vi "Measure Y verses voltage.vi"() -> ()   [LabVIEW 2020]
uses:
  <vilib>/DAQmx/write.llb/DAQmx Write (Analog 2D DBL NChan NSamp).vi
  <vilib>/DAQmx/create/channels.llb/DAQmx Create Channel (AO-Voltage-Basic).vi
  <vilib>/DAQmx/configure/timing.llb/DAQmx Timing (Use Waveform).vi
  <vilib>/Utility/file.llb/Write Delimited Spreadsheet (DBL).vi
  <vilib>/DAQmx/miscellaneous.llb/DAQmx Fill In Error Info.vi
  <vilib>/measure/NI_MABase.lvlib
panel:
  out "x+y":dbl=491.0
  in  "Voltage value at top of FOV":dbl=0.207
  out "dt":dbl=10.0
  out "Voice coil response (blue) 2":dbl[][](graph)=[[-0.284, -0.27908999999999995, -0.27418, -0.26927, -0.26436000000000004, -0.25945, -0.25454, -0.24963, -0.24472, -0.23981, -0.2349, -0.22999, -0.22507999999999997, -0.22017, -0.21525999999999998, -0.21034999999999998, -0.20544, -0.20053, -0.19562000000000002, -0.19071, -0.18580000000000002, -0.18089, -0.17598, -0.17107, -0.16616, -0.16125, -0.15634, -0.15143, -0.14651999999999998, -0.14160999999999999, -0.1367, -0.13179, -0.12688, -0.12197, -0.11706, -0.11215, -0.10724000000000002, -0.10232999999999999, -0.09741999999999999, -0.09251, -0.0876, -0.08269, -0.07778, -0.07287, -0.06795999999999998, -0.06304999999999998, -0.05813999999999998, -0.05322999999999999, -0.048319999999999995, -0.04341, -0.0385, -0.03359, -0.028680000000000008, -0.023769999999999982, -0.018860000000000012, -0.013949999999999988, -0.009039999999999963, -0.004129999999999996, 0.0007800000000000296, 0.005689999999999998, 0.010600000000000023, 0.01550999999999999, 0.020420000000000015, 0.025329999999999984, 0.03024000000000001, 0.035150000000000035, 0.040060000000000005, 0.044970000000000024, 0.049879999999999994, 0.05479000000000002, 0.05969999999999999, 0.06461000000000001, 0.06951999999999998, 0.07443000000000001, 0.07934000000000004, 0.08425, 0.08916000000000003, 0.09406999999999999, 0.09898000000000001, 0.10388999999999998, 0.10880000000000001, 0.11371000000000003, 0.11862, 0.12353000000000003, 0.12844, 0.13335000000000002, 0.13826, 0.14317000000000002, 0.14808000000000004, 0.15299000000000001, 0.15790000000000004, 0.16281, 0.16772000000000004, 0.17263, 0.17754000000000003, 0.18245, 0.18736000000000003, 0.19227000000000005, 0.19718, 0.20209000000000002, 0.207, 0.0, 0.0, 0.0, 0.0, 0.0, 0.0, 0.0, 0.0, 0.0, 0.0, 0.0, 0.0, 0.0, 0.0, 0.0, 0.0, 0.0, 0.0, 0.0, 0.0, 0.0, 0.0, 0.0, 0.0, 0.0, 0.0, 0.0, 0.0, 0.0, 0.0, 0.0, 0.0, 0.0, 0.0, 0.0, 0.0, 0.0, 0.0, 0.0, 0.0, 0.0, 0.0, 0.0, 0.0, 0.0, 0.0, 0.0, 0.0, 0.0, 0.0, 0.0, 0.0, 0.0, 0.0, 0.0, 0.0, 0.0, 0.0, 0.0, 0.0, 0.0, 0.0, 0.0, 0.0, 0.0, 0.0, 0.0, 0.0, 0.0, 0.0, 0.0, 0.0, 0.0, 0.0, 0.0, 0.0, 0.0, 0.0, 0.0, 0.0, 0.0, 0.0, 0.0, 0.0, 0.0, 0.0, 0.0, 0.0, 0.0, 0.0, 0.0, 0.0, 0.0, 0.0, 0.0, 0.0, 0.0, 0.0, 0.0, 0.0, 0.0, 0.0, 0.0, 0.0, 0.0, 0.0, 0.0, 0.0, 0.0, 0.0, 0.0, 0.0, 0.0, 0.0, 0.0, 0.0, 0.0, 0.0, 0.0, 0.0, 0.0, 0.0, 0.0, 0.0, 0.0, 0.0, 0.0, 0.0, 0.0, 0.0, 0.0, 0.0, 0.0, 0.0, 0.0, 0.0, 0.0, 0.0, 0.0, 0.0, 0.0, 0.0, 0.0, 0.0, 0.0, 0.0, 0.0, 0.0, 0.0, 0.0, 0.0, 0.0, 0.0, 0.0, 0.0, 0.0, 0.0, 0.0, 0.0, 0.0, 0.0, 0.0, 0.0, 0.0, 0.0, 0.0, 0.0, 0.0, 0.0, 0.0, 0.0, 0.0, 0.0, 0.0, 0.0, 0.0, 0.0, 0.0, 0.0, 0.0, 0.0, 0.0, 0.0, 0.0, 0.0, 0.0, 0.0, 0.0, 0.0, 0.0, 0.0, 0.0, 0.0, 0.0, 0.0, 0.0, 0.0, 0.0, 0.0, 0.0, 0.0, 0.0, 0.0, 0.0, 0.0, 0.0, 0.0, 0.0, 0.0, 0.0, 0.0, 0.0, 0.0, 0.0, 0.0, 0.0, 0.0, 0.0, 0.0, 0.0, 0.0, 0.0, 0.0, 0.0, 0.0, 0.0, 0.0, 0.0, 0.0, 0.0, 0.0, 0.0, 0.0, 0.0, 0.0, 0.0, 0.0, 0.0, 0.0, 0.0, 0.0, 0.0, 0.0, 0.0, 0.0, 0.0, 0.0, 0.0, 0.0, 0.0, 0.0, 0.0, 0.0, 0.0, 0.0, 0.0, 0.0, 0.0, 0.0, 0.0, 0.0, 0.0, 0.0, 0.0, 0.0, 0.0, 0.0, 0.0, 0.0, 0.0, 0.0, 0.0, 0.0, 0.0, 0.0, 0.0, 0.0, 0.0, 0.0, 0.0, 0.0, 0.0, 0.0, 0.0, 0.0, 0.0, 0.0, 0.0, 0.0, 0.0, 0.0, 0.0, 0.0, 0.0, 0.0, 0.0, 0.0, 0.0, 0.0, 0.0, 0.0, 0.0, 0.0, 0.0, 0.0, 0.0, 0.0, 0.0, 0.0, 0.0, 0.0, 0.0, 0.0, 0.0, 0.0, 0.0, 0.0, 0.0, 0.0, 0.0, 0.0, 0.0, 0.0, 0.0, 0.0, 0.0, 0.0, 0.0, 0.0, 0.0, 0.0, 0.0, 0.0, 0.0, 0.0, 0.0, 0.0, 0.0, 0.0, 0.0, 0.0, 0.0, 0.0, 0.0, 0.0, 0.0, 0.0, 0.0, 0.0, 0.0, 0.0, 0.0, 0.0, 0.0, 0.0, 0.0, 0.0, 0.0, 0.0, 0.0, 0.0, 0.0, 0.0, 0.0, 0.0, 0.0, 0.0, 0.0, 0.0, 0.0, 0.0, 0.0, 0.0, 0.0, 0.0, 0.0, 0.0, 0.0, 0.0, 0.0, 0.0, 0.0, 0.0, 0.0, 0.0, 0.0, 0.0, 0.0, 0.0, 0.0, 0.0, 0.0, 0.0, 0.0, 0.0, 0.0, 0.0, 0.0, 0.0, 0.0, 0.0, 0.0, 0.0, 0.0, 0.0, 0.0, 0.0, 0.0, 0.0, 0.0, 0.0, 0.0, 0.0, 0.0, 0.0, 0.0, 0.0, 0.0, 0.0, 0.0, 0.0, 0.0, 0.0, 0.0, 0.0, 0.0, 0.0, 0.0, 0.0, 0.0, 0.0, 0.0, 0.0, 0.0, 0.0, 0.0, 0.0, 0.0, 0.0, 0.0, 0.0, 0.0, 0.0, 0.0, 0.0, 0.0, 0.0, 0.0, 0.0, 0.0, 0.0, 0.0, 0.0, 0.0, 0.0, 0.0, 0.0, 0.0, 0.0, 0.0, 0.0, 0.0, 0.0, 0.0, 0.0, 0.0, 0.0, 0.0, 0.0, 0.0, 0.0, 0.0, 0.0, 0.0, 0.0, 0.0, 0.0, 0.0, 0.0, 0.0, 0.0, 0.0, 0.0, 0.0, 0.0, 0.0, 0.0, 0.0, 0.0, 0.0, 0.0, 0.0, 0.0, 0.0, 0.0, 0.0, 0.0, 0.0, 0.0, 0.0, 0.0, 0.0, 0.0, 0.0, 0.0, 0.0, 0.0, 0.0, 0.0, 0.0, 0.0, 0.0, 0.0, 0.0, 0.0, 0.0, 0.0, 0.0, 0.0, 0.0, 0.0, 0.0, 0.0, 0.0, 0.0, 0.0, 0.0, 0.0, 0.0, 0.0, 0.0, 0.0, 0.0, 0.0, 0.0, 0.0, 0.0, 0.0, 0.0, 0.0, 0.0, 0.0, 0.0, 0.0, 0.0, 0.0, 0.0, 0.0, 0.0, 0.0, 0.0, 0.0, 0.0, 0.0, 0.0, 0.0, 0.0, 0.0, 0.0, 0.0, 0.0, 0.0, 0.0, 0.0, 0.0, 0.0, 0.0, 0.0, 0.0, 0.0, 0.0, 0.0, 0.0, 0.0, 0.0, 0.0, 0.0, 0.0, 0.0, 0.0, 0.0, 0.0, 0.0, 0.0, 0.0, 0.0, 0.0, 0.0, 0.0, 0.0, 0.0, 0.0, 0.0, 0.0, 0.0, 0.0, 0.0, 0.0, 0.0, 0.0, 0.0, 0.0, 0.0, 0.0, 0.0, 0.0, 0.0, 0.0, 0.0, 0.0, 0.0, 0.0, 0.0, 0.0, 0.0, 0.0, 0.0, 0.0, 0.0, 0.0, 0.0, 0.0, 0.0, 0.0, 0.0, 0.0, 0.0, 0.0, 0.0, 0.0, 0.0, 0.0, 0.0, 0.0, 0.0, 0.0, 0.0, 0.0, 0.0, 0.0, 0.0, 0.0, 0.0, 0.0, 0.0, 0.0, 0.0, 0.0, 0.0, 0.0, 0.0, 0.0, 0.0, 0.0, 0.0, 0.0, 0.0, 0.0, 0.0, 0.0, 0.0, 0.0, 0.0, 0.0, 0.0, 0.0, 0.0, 0.0, 0.0, 0.0, 0.0, 0.0, 0.0, 0.0, 0.0, 0.0, 0.0, 0.0, 0.0, 0.0, 0.0, 0.0, 0.0, 0.0, 0.0, 0.0, 0.0, 0.0, 0.0, 0.0, 0.0, 0.0, 0.0, 0.0, 0.0, 0.0, 0.0, 0.0, 0.0, 0.0, 0.0, 0.0, 0.0, 0.0, 0.0, 0.0, 0.0, 0.0, 0.0, 0.0, 0.0, 0.0, 0.0, 0.0, 0.0, 0.0, 0.0, 0.0, 0.0, 0.0, 0.0, 0.0, 0.0, 0.0, 0.0, 0.0, 0.0, 0.0, 0.0, 0.0, 0.0, 0.0, 0.0, 0.0, 0.0, 0.0, 0.0, 0.0, 0.0, 0.0, 0.0, 0.0, 0.0, 0.0, 0.0, 0.0, 0.0, 0.0, 0.0, 0.0, 0.0, 0.0, 0.0, 0.0, 0.0, 0.0, 0.0, 0.0, 0.0, 0.0, 0.0, 0.0, 0.0, 0.0, 0.0, 0.0, 0.0, 0.0, 0.0, 0.0, 0.0, 0.0, 0.0, 0.0, 0.0, 0.0, 0.0, 0.0, 0.0, 0.0, 0.0, 0.0, 0.0, 0.0, 0.0, 0.0, 0.0, 0.0, 0.0, 0.0, 0.0, 0.0, 0.0, 0.0, 0.0, 0.0, 0.0, 0.0, 0.0, 0.0, 0.0, 0.0, 0.0, 0.0, 0.0, 0.0, 0.0, 0.0, 0.0, 0.0, 0.0, 0.0, 0.0, 0.0, 0.0, 0.0, 0.0, 0.0, 0.0, 0.0, 0.0, 0.0, 0.0, 0.0, 0.0, 0.0, 0.0, 0.0, 0.0, 0.0, 0.0, 0.0, 0.0, 0.0, 0.0, 0.0, 0.0, 0.0, 0.0, 0.0, 0.0, 0.0, 0.0, 0.0, 0.0, 0.0, 0.0, 0.0, 0.0, 0.0, 0.0, 0.0, 0.0, 0.0, 0.0, 0.0, 0.0, 0.0, 0.0, 0.0, 0.0, 0.0, 0.0, 0.0, 0.0, 0.0, 0.0, 0.0, 0.0, 0.0, 0.0, 0.0, 0.0, 0.0, 0.0, 0.0, 0.0, 0.0, 0.0, 0.0, 0.0, 0.0, 0.0, 0.0, 0.0, 0.0, 0.0, 0.0, 0.0, 0.0, 0.0, 0.0, 0.0, 0.0, 0.0, 0.0, 0.0, 0.0, 0.0], [0.0, 5.0, 0.0, 5.0, 0.0, 5.0, 0.0, 5.0, 0.0, 5.0, 0.0, 5.0, 0.0, 5.0, 0.0, 5.0, 0.0, 5.0, 0.0, 5.0, 0.0, 5.0, 0.0, 5.0, 0.0, 5.0, 0.0, 5.0, 0.0, 5.0, 0.0, 5.0, 0.0, 5.0, 0.0, 5.0, 0.0, 5.0, 0.0, 5.0, 0.0, 5.0, 0.0, 5.0, 0.0, 5.0, 0.0, 5.0, 0.0, 5.0, 0.0, 5.0, 0.0, 5.0, 0.0, 5.0, 0.0, 5.0, 0.0, 5.0, 0.0, 5.0, 0.0, 5.0, 0.0, 5.0, 0.0, 5.0, 0.0, 5.0, 0.0, 5.0, 0.0, 5.0, 0.0, 5.0, 0.0, 5.0, 0.0, 5.0, 0.0, 5.0, 0.0, 5.0, 0.0, 5.0, 0.0, 5.0, 0.0, 5.0, 0.0, 5.0, 0.0, 5.0, 0.0, 5.0, 0.0, 5.0, 0.0, 5.0, 0.0, 5.0, 0.0, 5.0, 0.0, 5.0, 0.0, 5.0, 0.0, 5.0, 0.0, 5.0, 0.0, 5.0, 0.0, 5.0, 0.0, 5.0, 0.0, 5.0, 0.0, 5.0, 0.0, 5.0, 0.0, 5.0, 0.0, 5.0, 0.0, 5.0, 0.0, 5.0, 0.0, 5.0, 0.0, 5.0, 0.0, 5.0, 0.0, 5.0, 0.0, 5.0, 0.0, 5.0, 0.0, 5.0, 0.0, 5.0, 0.0, 5.0, 0.0, 5.0, 0.0, 5.0, 0.0, 5.0, 0.0, 5.0, 0.0, 5.0, 0.0, 5.0, 0.0, 5.0, 0.0, 5.0, 0.0, 5.0, 0.0, 5.0, 0.0, 5.0, 0.0, 5.0, 0.0, 5.0, 0.0, 5.0, 0.0, 5.0, 0.0, 5.0, 0.0, 5.0, 0.0, 5.0, 0.0, 5.0, 0.0, 5.0, 0.0, 5.0, 0.0, 5.0, 0.0, 5.0, 0.0, 5.0, 0.0, 5.0, 0.0, 5.0, 0.0, 5.0, 0.0, 5.0, 0.0, 5.0, 0.0, 5.0, 0.0, 5.0, 0.0, 5.0, 0.0, 5.0, 0.0, 5.0, 0.0, 5.0, 0.0, 5.0, 0.0, 5.0, 0.0, 5.0, 0.0, 5.0, 0.0, 5.0, 0.0, 5.0, 0.0, 5.0, 0.0, 5.0, 0.0, 5.0, 0.0, 5.0, 0.0, 5.0, 0.0, 5.0, 0.0, 5.0, 0.0, 5.0, 0.0, 5.0, 0.0, 5.0, 0.0, 5.0, 0.0, 5.0, 0.0, 5.0, 0.0, 5.0, 0.0, 5.0, 0.0, 5.0, 0.0, 5.0, 0.0, 5.0, 0.0, 5.0, 0.0, 5.0, 0.0, 5.0, 0.0, 5.0, 0.0, 5.0, 0.0, 5.0, 0.0, 5.0, 0.0, 5.0, 0.0, 5.0, 0.0, 5.0, 0.0, 5.0, 0.0, 5.0, 0.0, 5.0, 0.0, 5.0, 0.0, 5.0, 0.0, 5.0, 0.0, 5.0, 0.0, 5.0, 0.0, 5.0, 0.0, 5.0, 0.0, 5.0, 0.0, 5.0, 0.0, 5.0, 0.0, 5.0, 0.0, 5.0, 0.0, 5.0, 0.0, 5.0, 0.0, 5.0, 0.0, 5.0, 0.0, 5.0, 0.0, 5.0, 0.0, 5.0, 0.0, 5.0, 0.0, 5.0, 0.0, 5.0, 0.0, 5.0, 0.0, 5.0, 0.0, 5.0, 0.0, 5.0, 0.0, 5.0, 0.0, 5.0, 0.0, 5.0, 0.0, 5.0, 0.0, 5.0, 0.0, 5.0, 0.0, 5.0, 0.0, 5.0, 0.0, 5.0, 0.0, 5.0, 0.0, 5.0, 0.0, 5.0, 0.0, 5.0, 0.0, 5.0, 0.0, 5.0, 0.0, 5.0, 0.0, 5.0, 0.0, 5.0, 0.0, 5.0, 0.0, 5.0, 0.0, 5.0, 0.0, 5.0, 0.0, 5.0, 0.0, 5.0, 0.0, 5.0, 0.0, 5.0, 0.0, 5.0, 0.0, 5.0, 0.0, 5.0, 0.0, 5.0, 0.0, 5.0, 0.0, 5.0, 0.0, 5.0, 0.0, 5.0, 0.0, 5.0, 0.0, 5.0, 0.0, 5.0, 0.0, 5.0, 0.0, 5.0, 0.0, 5.0, 0.0, 5.0, 0.0, 5.0, 0.0, 5.0, 0.0, 5.0, 0.0, 5.0, 0.0, 5.0, 0.0, 5.0, 0.0, 5.0, 0.0, 5.0, 0.0, 5.0, 0.0, 5.0, 0.0, 5.0, 0.0, 5.0, 0.0, 5.0, 0.0, 5.0, 0.0, 5.0, 0.0, 5.0, 0.0, 5.0, 0.0, 5.0, 0.0, 5.0, 0.0, 5.0, 0.0, 5.0, 0.0, 5.0, 0.0, 5.0, 0.0, 5.0, 0.0, 5.0, 0.0, 5.0, 0.0, 5.0, 0.0, 5.0, 0.0, 5.0, 0.0, 5.0, 0.0, 5.0, 0.0, 5.0, 0.0, 5.0, 0.0, 5.0, 0.0, 5.0, 0.0, 5.0, 0.0, 5.0, 0.0, 5.0, 0.0, 5.0, 0.0, 5.0, 0.0, 5.0, 0.0, 5.0, 0.0, 5.0, 0.0, 5.0, 0.0, 5.0, 0.0, 5.0, 0.0, 5.0, 0.0, 5.0, 0.0, 5.0, 0.0, 5.0, 0.0, 5.0, 0.0, 5.0, 0.0, 5.0, 0.0, 5.0, 0.0, 5.0, 0.0, 5.0, 0.0, 5.0, 0.0, 5.0, 0.0, 5.0, 0.0, 5.0, 0.0, 5.0, 0.0, 5.0, 0.0, 5.0, 0.0, 5.0, 0.0, 5.0, 0.0, 5.0, 0.0, 5.0, 0.0, 5.0, 0.0, 5.0, 0.0, 5.0, 0.0, 5.0, 0.0, 5.0, 0.0, 5.0, 0.0, 5.0, 0.0, 5.0, 0.0, 5.0, 0.0, 5.0, 0.0, 5.0, 0.0, 5.0, 0.0, 5.0, 0.0, 5.0, 0.0, 5.0, 0.0, 5.0, 0.0, 5.0, 0.0, 5.0, 0.0, 5.0, 0.0, 5.0, 0.0, 5.0, 0.0, 5.0, 0.0, 5.0, 0.0, 5.0, 0.0, 5.0, 0.0, 5.0, 0.0, 5.0, 0.0, 5.0, 0.0, 5.0, 0.0, 5.0, 0.0, 5.0, 0.0, 5.0, 0.0, 5.0, 0.0, 5.0, 0.0, 5.0, 0.0, 5.0, 0.0, 5.0, 0.0, 5.0, 0.0, 5.0, 0.0, 5.0, 0.0, 5.0, 0.0, 5.0, 0.0, 5.0, 0.0, 5.0, 0.0, 5.0, 0.0, 5.0, 0.0, 5.0, 0.0, 5.0, 0.0, 5.0, 0.0, 5.0, 0.0, 5.0, 0.0, 5.0, 0.0, 5.0, 0.0, 5.0, 0.0, 5.0, 0.0, 5.0, 0.0, 5.0, 0.0, 5.0, 0.0, 5.0, 0.0, 5.0, 0.0, 5.0, 0.0, 5.0, 0.0, 5.0, 0.0, 5.0, 0.0, 5.0, 0.0, 5.0, 0.0, 5.0, 0.0, 5.0, 0.0, 5.0, 0.0, 5.0, 0.0, 5.0, 0.0, 5.0, 0.0, 5.0, 0.0, 5.0, 0.0, 5.0, 0.0, 5.0, 0.0, 5.0, 0.0, 5.0, 0.0, 5.0, 0.0, 5.0, 0.0, 5.0, 0.0, 5.0, 0.0, 5.0, 0.0, 5.0, 0.0, 5.0, 0.0, 5.0, 0.0, 5.0, 0.0, 5.0, 0.0, 5.0, 0.0, 5.0, 0.0, 5.0, 0.0, 5.0, 0.0, 5.0, 0.0, 5.0, 0.0, 5.0, 0.0, 5.0, 0.0, 5.0, 0.0, 5.0, 0.0, 5.0, 0.0, 5.0, 0.0, 5.0, 0.0, 5.0, 0.0, 5.0, 0.0, 5.0, 0.0, 5.0, 0.0, 5.0, 0.0, 5.0, 0.0, 5.0, 0.0, 5.0, 0.0, 5.0, 0.0, 5.0, 0.0, 5.0, 0.0, 5.0, 0.0, 5.0, 0.0, 5.0, 0.0, 5.0, 0.0, 5.0, 0.0, 5.0, 0.0, 5.0, 0.0, 5.0, 0.0, 5.0, 0.0, 5.0, 0.0, 5.0, 0.0, 5.0, 0.0, 5.0, 0.0, 5.0, 0.0, 5.0, 0.0, 5.0, 0.0, 5.0, 0.0, 5.0, 0.0, 5.0, 0.0, 5.0, 0.0, 5.0, 0.0, 5.0, 0.0, 5.0, 0.0, 5.0, 0.0, 5.0, 0.0, 5.0, 0.0, 5.0, 0.0, 5.0, 0.0, 5.0, 0.0, 5.0, 0.0, 5.0, 0.0, 5.0, 0.0, 5.0, 0.0, 5.0, 0.0, 5.0, 0.0, 5.0, 0.0, 5.0, 0.0, 5.0, 0.0, 5.0, 0.0, 5.0, 0.0, 5.0, 0.0, 5.0, 0.0, 5.0, 0.0, 5.0, 0.0, 5.0, 0.0, 5.0, 0.0, 5.0, 0.0, 5.0, 0.0, 5.0, 0.0, 5.0, 0.0, 5.0, 0.0, 5.0, 0.0, 5.0, 0.0, 5.0, 0.0, 5.0, 0.0, 5.0, 0.0, 5.0, 0.0, 5.0, 0.0, 5.0, 0.0, 5.0, 0.0, 5.0, 0.0, 5.0, 0.0, 5.0, 0.0, 5.0, 0.0, 5.0, 0.0, 5.0, 0.0, 5.0, 0.0, 5.0, 0.0, 5.0, 0.0, 5.0, 0.0, 5.0, 0.0, 5.0, 0.0, 5.0, 0.0, 5.0, 0.0, 5.0, 0.0, 5.0, 0.0, 5.0, 0.0, 5.0, 0.0, 5.0, 0.0, 5.0, 0.0, 5.0, 0.0, 5.0, 0.0, 5.0, 0.0, 5.0, 0.0, 5.0, 0.0, 5.0, 0.0, 5.0, 0.0, 5.0, 0.0, 5.0, 0.0, 5.0, 0.0, 5.0, 0.0, 5.0, 0.0, 5.0, 0.0, 5.0, 0.0, 5.0, 0.0, 5.0, 0.0, 5.0, 0.0, 5.0, 0.0, 5.0, 0.0, 5.0, 0.0, 5.0, 0.0, 5.0, 0.0, 5.0, 0.0, 5.0, 0.0, 5.0, 0.0, 5.0, 0.0, 5.0]]
  out "x/y 2":dbl=0.01
  out "x/y":dbl=4.91
  out "x*y":dbl=491.0
  in  "Number of frames":dbl=100.0
  in  "file path (dialog if empty)":path=path "C:/Users/htm22/Downloads/Voltage positions.txt"
  in  "Voltage value at bottom of FOV":dbl=-0.284
  out "# Samples written per channel":u32=1000
  in  "Stop 2":bool
  out "Maximum Voltage value at top of FOV":dbl=0.207
  out "Voice coil response (blue)":waveform(dbl)[](graph)=[{"t0"=timestamp(0 s since 1904-01-01), "dt"=10.0, "Y"=[-0.284, -0.27908999999999995, -0.27418, -0.26927, -0.26436000000000004, -0.25945, -0.25454, -0.24963, -0.24472, -0.23981, -0.2349, -0.22999, -0.22507999999999997, -0.22017, -0.21525999999999998, -0.21034999999999998, -0.20544, -0.20053, -0.19562000000000002, -0.19071, -0.18580000000000002, -0.18089, -0.17598, -0.17107, -0.16616, -0.16125, -0.15634, -0.15143, -0.14651999999999998, -0.14160999999999999, -0.1367, -0.13179, -0.12688, -0.12197, -0.11706, -0.11215, -0.10724000000000002, -0.10232999999999999, -0.09741999999999999, -0.09251, -0.0876, -0.08269, -0.07778, -0.07287, -0.06795999999999998, -0.06304999999999998, -0.05813999999999998, -0.05322999999999999, -0.048319999999999995, -0.04341, -0.0385, -0.03359, -0.028680000000000008, -0.023769999999999982, -0.018860000000000012, -0.013949999999999988, -0.009039999999999963, -0.004129999999999996, 0.0007800000000000296, 0.005689999999999998, 0.010600000000000023, 0.01550999999999999, 0.020420000000000015, 0.025329999999999984, 0.03024000000000001, 0.035150000000000035, 0.040060000000000005, 0.044970000000000024, 0.049879999999999994, 0.05479000000000002, 0.05969999999999999, 0.06461000000000001, 0.06951999999999998, 0.07443000000000001, 0.07934000000000004, 0.08425, 0.08916000000000003, 0.09406999999999999, 0.09898000000000001, 0.10388999999999998, 0.10880000000000001, 0.11371000000000003, 0.11862, 0.12353000000000003, 0.12844, 0.13335000000000002, 0.13826, 0.14317000000000002, 0.14808000000000004, 0.15299000000000001, 0.15790000000000004, 0.16281, 0.16772000000000004, 0.17263, 0.17754000000000003, 0.18245, 0.18736000000000003, 0.19227000000000005, 0.19718, 0.20209000000000002, 0.207]}, {"t0"=timestamp(0 s since 1904-01-01), "dt"=10.0, "Y"=array[1000 elements]}]
  # "Fs= sampling rate in samples per second\n#s= number of samples in the waveform"
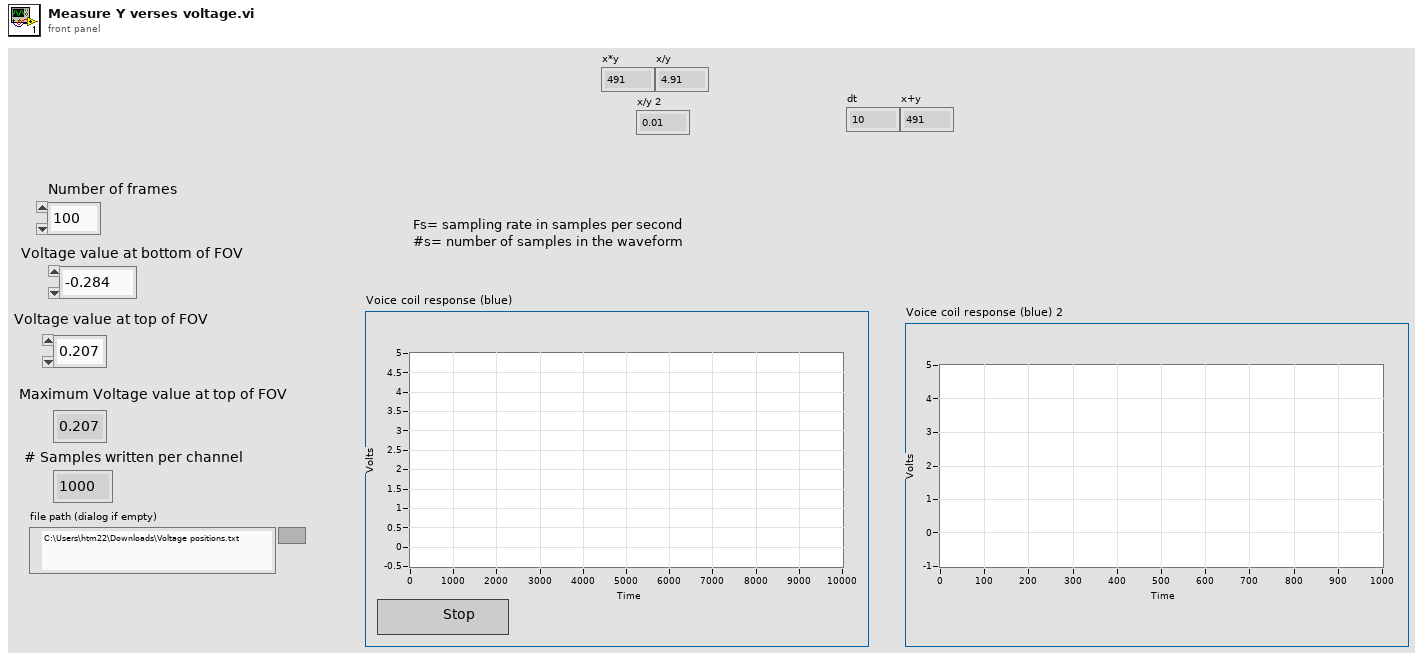
[diagram p1: front panel]
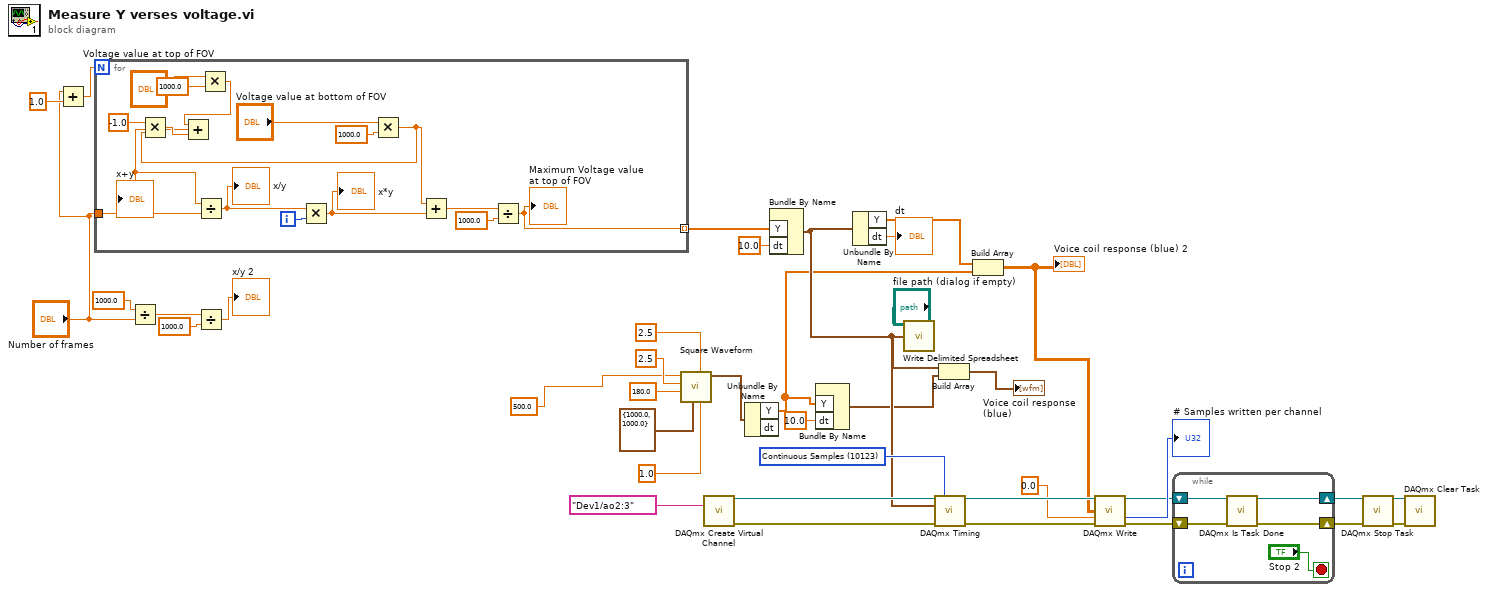
[diagram p0: block diagram]
diagram:
  w37 = 10123 items=["Finite Samples"=10178, "Continuous Samples"=10123, "Hardware Timed Single Point"=12522] ("sample mode")
  n1 = Add(x="Number of frames", y=1.0) -> (x+y=w13:dbl)
  n2 = for {
    N: w13 -> [_]
    tunnel: [w47] -> w10 mode=indexing
    tunnel: "Number of frames" -> [w54]
    i -> [w55]
    n3 = Multiply(x="Voltage value at top of FOV", y=1000.0) -> (x*y=w43:dbl)
    n4 = Multiply(x="Voltage value at bottom of FOV", y=1000.0) -> (x*y=w45:dbl)
    n5 = Multiply(x=-1.0, y=w45) -> (x*y=w44:dbl)
    n6 = Add(x=w43, y=w44) -> (x+y=w40:dbl)
    "x+y" <- w40
    n7 = Divide(x=w40, y=w54) -> (x/y=w52:dbl)
    "x/y" <- w52
    n8 = Multiply(x=w52, y=w55) -> (x*y=w53:dbl)
    "x*y" <- w53
    n9 = Add(x=w45, y=w53) -> (x+y=w48:dbl)
    n10 = Divide(x=w48, y=1000.0) -> (x/y=w47:dbl)
    "Maximum Voltage value at top of FOV" <- w47
  }
  n11 = Divide(x=1000.0, y="Number of frames") -> (x/y=w17:dbl)
  n12 = Divide(x=w17, y=1000.0) -> (x/y=→"x/y 2":dbl)
  n13 = call <vilib>:"Square Waveform.vi"("duty cycle (%)"=1.0, "offset"=2.5, "sampling info"=cluster{"Fs":dbl, "#s":dbl} {"Fs"=1000.0, "#s"=1000.0}, "phase"=180.0, "amplitude"=2.5, "frequency"=500.0) -> ("signal out"=w9:waveform(dbl))  [unwired: 4 in, 1 out]
  n14 = call-poly <vilib>:"DAQmx Create Virtual Channel.vi"("physical channels"=tag "Dev1/ao2:3") -> ("task out"=w39:refnum<k21>, "error out"=w38:errorcluster)  [unwired: 13 in]
  n15 = Unbundle By Name(w9) -> ("Y"=w3:dbl[])  [unwired: 1 out]
  n16 = Bundle By Name("Y"=w10, "dt"=10.0) -> (w8:waveform(dbl))  [unwired: 1 in]
  n17 = Bundle By Name("Y"=w3, "dt"=10.0) -> (w1:waveform(dbl))  [unwired: 1 in]
  n18 = Unbundle By Name(w8) -> ("Y"=w6:dbl[], "dt"=→"dt":dbl)
  n19 = call-poly <vilib>:"Write Delimited Spreadsheet.vi"("file path (dialog if empty)"="file path (dialog if empty)", "1D data"=w8) -> ()  [unwired: 12 in, 2 out]
  n20 = call-poly <vilib>:"DAQmx Timing.vi"("task/channels in"=w39, "sample mode"=w37, "waveform"=w8, "error in"=w38) -> ("task out"=w26:refnum<k21>, "error out"=w36:errorcluster)  [unwired: 10 in]
  n21 = Build Array(w8, w1) -> (→"Voice coil response (blue)":waveform(dbl)[])
  n22 = Build Array(w6, w3) -> (w12:dbl[][])
  "Voice coil response (blue) 2" <- w12
  n23 = call-poly <vilib>:"DAQmx Write.vi"("task/channels in"=w26, "data"=w12, "timeout"=0.0, "error in"=w36) -> ("task out"=w29:refnum<k21>, "number of samples written per channel"=→"# Samples written per channel":u32, "error out"=w28:errorcluster)  [unwired: 9 in]
  n24 = while {
    shift-right: [w57] -> w31
    shift-left: w29 -> [w60]
    shift-right: [w58] -> w32
    shift-left: w28 -> [w59]
    stop <- "Stop 2" stop-if-true
    n25 = call <vilib>:"DAQmx Is Task Done.vi"("task/channels in"=w60, "error in"=w59) -> ("task out"=w57:refnum<k21>, "error out"=w58:errorcluster)  [unwired: 11 in, 1 out]
  }
  n26 = call <vilib>:"DAQmx Stop Task.vi"("task/channels in"=w31, "error in"=w32) -> ("task out"=w33:refnum<k21>, "error out"=w34:errorcluster)  [unwired: 12 in]
  n27 = call <vilib>:"DAQmx Clear Task.vi"("task in"=w33, "error in"=w34) -> ()  [unwired: 13 in, 1 out]
